vi "PING RT.vi"(8 "错误输入（无错误）":errorcluster, 11 "引用句柄输入":refnum<k20> caption="Custom FPGA Reference Out") -> (0 "错误输出":errorcluster, 2 "PING":u32[](array[numeric]), 3 "引用句柄输出":refnum<k20> caption="FPGA VI引用输出")   [LabVIEW 2017]
uses:
  <vilib>/Utility/error.llb/Error Cluster From Error Code.vi
  <vilib>/rvi/errors/niLvFpgaAdjustHostInterfaceError.vi
  <vilib>/rvi/interface/nirviReadWriteControl/nirviReadWriteControl.xnode
  NiFpgaLv.dll
  <vilib>/rvi/interface/Simulation/niFpgaSimulationCallBeginRW.vi
  <vilib>/ptbypt/NI_PtbyPt.lvlib
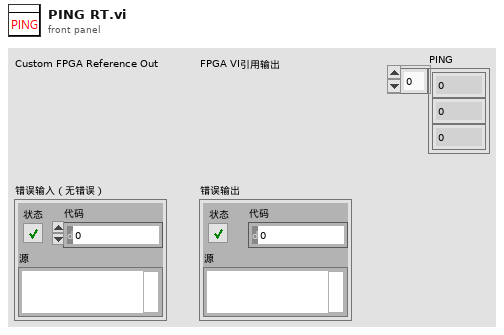
[diagram p1: front panel]
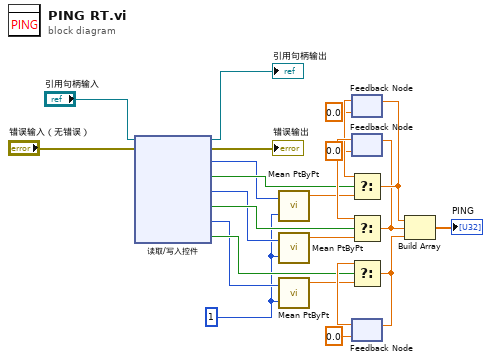
[diagram p0: block diagram]
diagram:
  w4 = 1 ("sample length")
  n1 = xnode "读取/写入控件"("FPGA VI引用输入"="引用句柄输入", "错误输入"="错误输入（无错误）") -> ("FPGA VI引用输出"=→"引用句柄输出":refnum<k20>, "错误输出"=→"错误输出":errorcluster, "PING1"=w12:u32, "timed out1"=w13:bool, "PING2"=w10:u32, "timed out2"=w15:bool, "PING3"=w8:u32, "timed out3"=w16:bool)
  n2 = call <vilib>:"Mean PtByPt.vi"("x"=w12, "sample length"=w4) -> ("mean"=w11:dbl)  [unwired: 2 in, 1 out]
  n3 = call <vilib>:"Mean PtByPt.vi"("x"=w10, "sample length"=w4) -> ("mean"=w9:dbl)  [unwired: 2 in, 1 out]
  n4 = call <vilib>:"Mean PtByPt.vi"("x"=w8, "sample length"=w4) -> ("mean"=w7:dbl)  [unwired: 2 in, 1 out]
  n5 = feedback #1(0.0 ("mean")) -> (w14:dbl)
  n6 = feedback #2(0.0 ("mean")) -> (w17:dbl)
  n7 = Select(t=w14, s=w13, f=w11) -> (s? t:f=w21:dbl)
  n8 = feedback-in #1(w21) -> ()
  n9 = Select(t=w17, s=w15, f=w9) -> (s? t:f=w20:dbl)
  n10 = feedback-in #2(w20) -> ()
  n11 = feedback #3(0.0 ("mean")) -> (w18:dbl)
  n12 = Select(t=w18, s=w16, f=w7) -> (s? t:f=w19:dbl)
  n13 = feedback-in #3(w19) -> ()
  n14 = Build Array(w21, w20, w19) -> (→"PING":dbl[])
